vi "Read TV.vi"(8 "error in (no error)":errorcluster, 11 "Keysight44xx in":refnum<class "Keysight44xx.lvclass">) -> (0 "error out":errorcluster, 2 "TV":T1={"Monitor Enabled (OFF)"=FALSE, "SynchronizeSweep"=FALSE, "SynchronizationLineNumber"=0, "TV Field (Any Field)"=3, "TV Signal Format (NTSC-M)"=1, "Trigger Source (Spectrum Analyzer)"=2} {"Trigger Source (Spectrum Analyzer)" items=["External"=1, "Spectrum Analyzer"=2]; "TV Signal Format (NTSC-M)" items=["NTSC-M"=1, "NTSC-Japan"=2, "PAL-M"=3, "PAL-B,D,G,H,I"=4, "PAL-N"=5, "PAL-N Combin"=6, "SECAM-L"=7]; "TV Field (Any Field)" items=["Field 1"=1, "Field 2"=2, "Any Field"=3]}, 3 "Keysight44xx out":refnum<class "Keysight44xx.lvclass">)   [LabVIEW 2018, in "SpecAnPlugins.lvlib" / "Keysight44xx.lvclass"]
uses:
  Keysight44xx.lvclass
  TypeDefs/TV.ctl
  Keysight44xx.lvclass/Keysight44xx.ctl
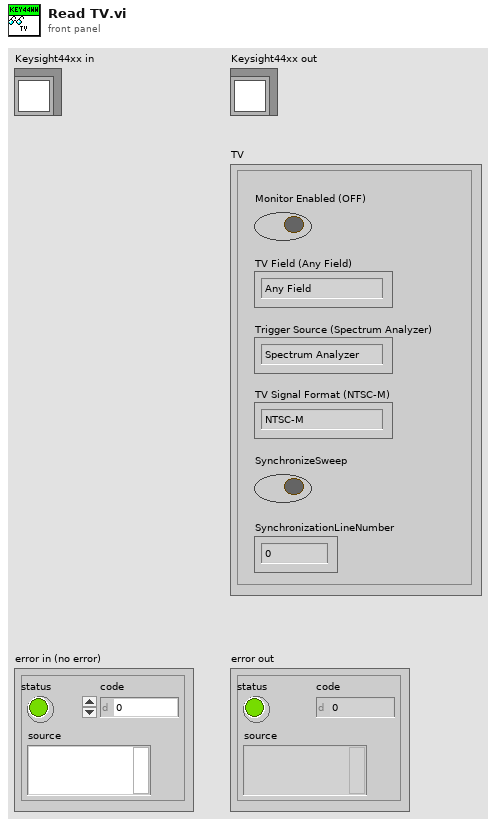
[diagram p1: front panel]
types:
  T1 = typedef "SpecAnPlugins.lvlib/Keysight44xx.lvclass/TV.ctl" = cluster{"Monitor Enabled (OFF)":bool, "SynchronizeSweep":bool, "SynchronizationLineNumber":i32, "TV Field (Any Field)":i32, "TV Signal Format (NTSC-M)":i32, "Trigger Source (Spectrum Analyzer)":i32}
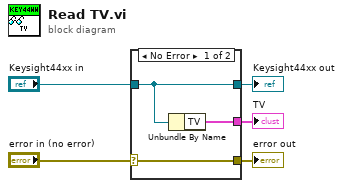
[diagram p0: block diagram]
diagram:
  n1 = case shown="No Error" "error in (no error)" {
    selector: "error in (no error)" -> [w8 w9]
    tunnel: [w8 w9] -> w4
    tunnel: [w7 w10] -> w2
    tunnel: "Keysight44xx in" -> [w7 w10]
    tunnel: [w6 _] -> w1
    frame No Error {
      n2 = Unbundle By Name(w7) -> ("TV"=w6:T1)
    }
    frame Error {
    }
  }
  "error out" <- w4
  "Keysight44xx out" <- w2
  "TV" <- w1
